vi "Read Errors Array.vi"(8 "error in (no error)":errorcluster, 11 "Simulated_CCD_Camera in":refnum<class "Simulated_CCD_Camera.lvclass">) -> (0 "error out":errorcluster, 2 "Errors array":errorcluster[](array[cluster]), 3 "Simulated_CCD_Camera out":refnum<class "Simulated_CCD_Camera.lvclass">)   [LabVIEW 2018, in "Simulated_CCD_Camera.lvclass"]
uses:
  Simulated_CCD_Camera.lvclass
  Simulated_CCD_Camera.lvclass/Simulated_CCD_Camera.ctl
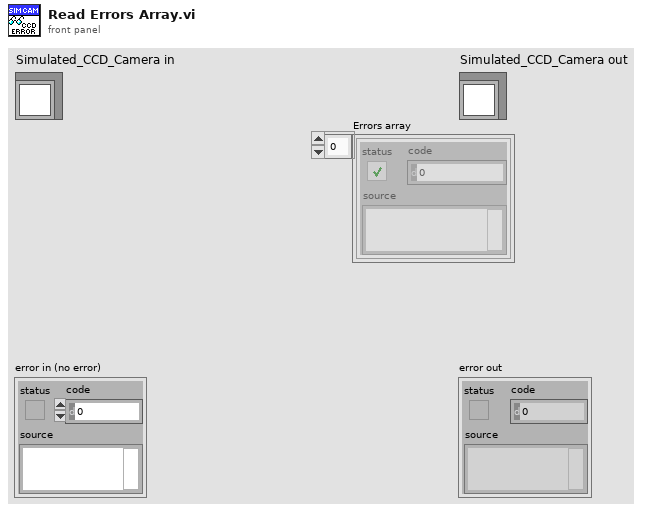
[diagram p1: front panel]
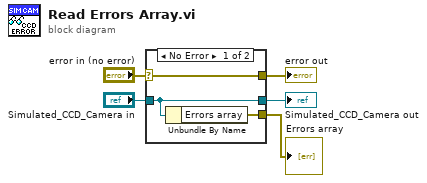
[diagram p0: block diagram]
diagram:
  n1 = case shown="No Error" "error in (no error)" {
    selector: "error in (no error)" -> [w7 w10]
    tunnel: "Simulated_CCD_Camera in" -> [w6 w9]
    tunnel: [w8 _] -> w1
    tunnel: [w7 w10] -> w3
    tunnel: [w6 w9] -> w2
    frame No Error {
      n2 = Unbundle By Name(w6) -> ("Errors array"=w8:errorcluster[])
    }
    frame Error {
    }
  }
  "error out" <- w3
  "Simulated_CCD_Camera out" <- w2
  "Errors array" <- w1
